vi "Erase and Write pulse control V1.1.vi"() -> ()   [LabVIEW 2016]
uses:
  <userlib>/LevyLab/Relay Box/Type_defs/Resistor--enum.ctl
panel:
  out "error out":errorcluster
  in  "error in":errorcluster
  in  "Set Resistance":T1=enum."1G ohm"
  in  "Z SetPoint: Lift the tip a little":dbl=-0.03 format="%#_6p"
  in  "Withdraw tip?":bool
  in  "wait time second pulse 3":u32=500
  in  "Second pulse 3":dbl=16.0 format="%_5p"
  in  "wait time between 3":u32=500
  in  "Wait time first pulse  2":u32=2000
  in  "First pulse 3":dbl=-15.0 format="%_5p"
  in  "Z SetPoint 3":dbl=-0.29 format="%#_6p"
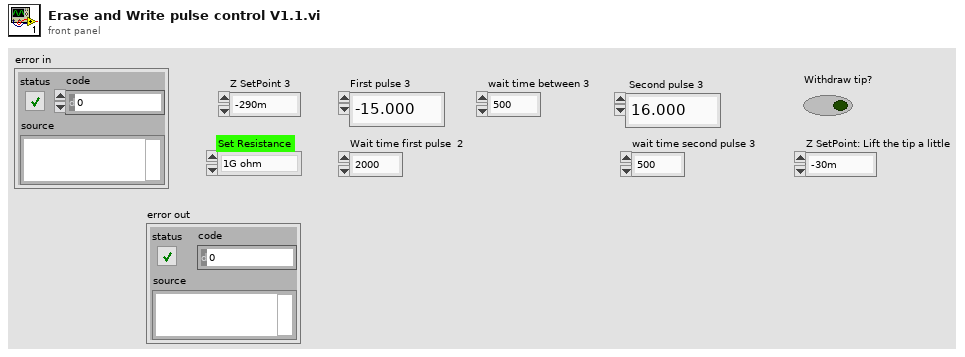
[diagram p1: front panel]
types:
  T1 = typedef "Resistor--enum.ctl" = enum16{"open", "discharge tip", "0 ohms", "100k ohm", "10M ohm", "1G ohm"}
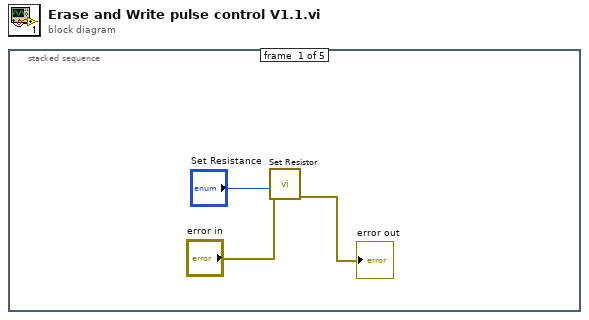
[diagram p0: block diagram]
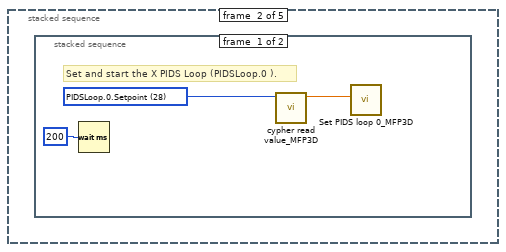
[diagram p2: hidden frame]
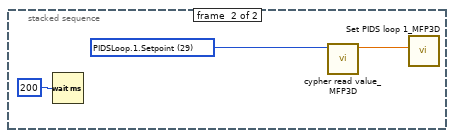
[diagram p3: hidden frame]
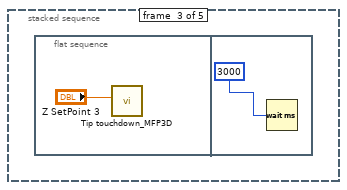
[diagram p4: hidden frame]
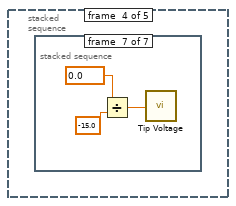
[diagram p5: hidden frame]
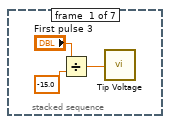
[diagram p6: hidden frame]
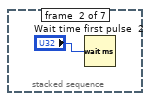
[diagram p7: hidden frame]
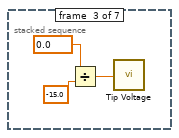
[diagram p8: hidden frame]
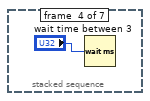
[diagram p9: hidden frame]
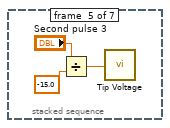
[diagram p10: hidden frame]
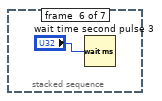
[diagram p11: hidden frame]
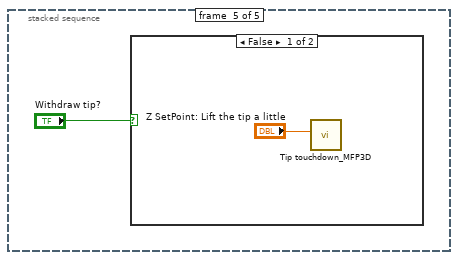
[diagram p12: hidden frame]
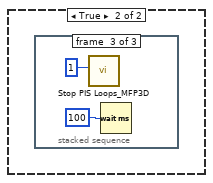
[diagram p13: hidden frame]
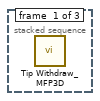
[diagram p14: hidden frame]
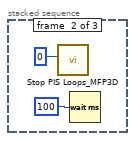
[diagram p15: hidden frame]
diagram:
  n1 = stacked-sequence {
    frame #0 {
      n2 = call <userlib>:"Set Resistor.vi"("error in"="error in", "Set Resistance"="Set Resistance") -> ("error out"=→"error out":errorcluster)  [unwired: 9 in]
    }
    frame #1 {
      n3 = stacked-sequence {
        frame #0 {
          w5 = u16 28 items=["XSensor", "YSensor", "ZSensor", "InA", "InB", "InFast", "In_Amplitude1", "In_Amplitude2", "In_Phase1", "In_Phase2", "PiezoX", "PiezoY", "PiezoZ", "OutA", "OutB", "OutC", "DDS_Frequency1", "DDS_Frequency2", "DDS_Amplitude1", "DDS_Amplitude2", "DDS_DCOffset", "Laser_Sum", "Laser_Difference", "Laser_Lateral", "XLVDT Sensitivity", "YLVDT Sensitivity", "XLVDT Offset", "YLVDT Offset", "PIDSLoop.0.Setpoint", "PIDSLoop.1.Setpoint"] ("Input")
          # "Set and start the X PIDS Loop (PIDSLoop.0 )."
          n4 = Wait (ms)(milliseconds to wait=u32 200) -> ()  [unwired: 1 out]
          n5 = call <vilib>:"cypher read value_MFP3D.vi"("Input"=w5) -> ("Result"=w6:dbl)  [unwired: 10 in]
          n6 = call <vilib>:"Set PIDS loop 0_MFP3D.vi"("X  Setpoint"=w6) -> ()  [unwired: 11 in]
        }
        frame #1 {
          w8 = u16 29 items=["XSensor", "YSensor", "ZSensor", "InA", "InB", "InFast", "In_Amplitude1", "In_Amplitude2", "In_Phase1", "In_Phase2", "PiezoX", "PiezoY", "PiezoZ", "OutA", "OutB", "OutC", "DDS_Frequency1", "DDS_Frequency2", "DDS_Amplitude1", "DDS_Amplitude2", "DDS_DCOffset", "Laser_Sum", "Laser_Difference", "Laser_Lateral", "XLVDT Sensitivity", "YLVDT Sensitivity", "XLVDT Offset", "YLVDT Offset", "PIDSLoop.0.Setpoint", "PIDSLoop.1.Setpoint"] ("Input")
          n7 = Wait (ms)(milliseconds to wait=u32 200) -> ()  [unwired: 1 out]
          n8 = call <vilib>:"cypher read value_MFP3D.vi"("Input"=w8) -> ("Result"=w7:dbl)  [unwired: 10 in]
          n9 = call <vilib>:"Set PIDS loop 1_MFP3D.vi"("Y Setpoint"=w7) -> ()  [unwired: 11 in]
        }
      }
    }
    frame #2 {
      n10 = flat-sequence {
        frame #0 {
          n11 = call <vilib>:"Tip touchdown_MFP3D.vi"("Z SetPoint"="Z SetPoint 3") -> ()  [unwired: 11 out]
        }
        frame #1 {
          n12 = Wait (ms)(milliseconds to wait=u32 3000 ("Wait time first pulse  2")) -> ()  [unwired: 1 out]
        }
      }
    }
    frame #3 {
      n13 = stacked-sequence {
        frame #0 {
          n14 = Divide(x="First pulse 3", y=-15.0) -> (x/y=w12:dbl)
          n15 = call <userlib>:"Tip Voltage.vi"("Output Voltage"=w12) -> ()  [unwired: 1 out]
        }
        frame #1 {
          n16 = Wait (ms)(milliseconds to wait="Wait time first pulse  2") -> ()  [unwired: 1 out]
        }
        frame #2 {
          n17 = Divide(x=0.0 ("Output Voltage 2"), y=-15.0) -> (x/y=w18:dbl)
          n18 = call <userlib>:"Tip Voltage.vi"("Output Voltage"=w18) -> ()  [unwired: 1 out]
        }
        frame #3 {
          n19 = Wait (ms)(milliseconds to wait="wait time between 3") -> ()  [unwired: 1 out]
        }
        frame #4 {
          n20 = Divide(x="Second pulse 3", y=-15.0) -> (x/y=w22:dbl)
          n21 = call <userlib>:"Tip Voltage.vi"("Output Voltage"=w22) -> ()  [unwired: 1 out]
        }
        frame #5 {
          n22 = Wait (ms)(milliseconds to wait="wait time second pulse 3") -> ()  [unwired: 1 out]
        }
        frame #6 {
          n23 = Divide(x=0.0 ("Output Voltage 2"), y=-15.0) -> (x/y=w26:dbl)
          n24 = call <userlib>:"Tip Voltage.vi"("Output Voltage"=w26) -> ()  [unwired: 1 out]
        }
      }
    }
    frame #4 {
      n25 = case shown="False" "Withdraw tip?" {
        frame False {
          n26 = call <vilib>:"Tip touchdown_MFP3D.vi"("Z SetPoint"="Z SetPoint: Lift the tip a little") -> ()  [unwired: 11 out]
        }
        frame True {
          n27 = stacked-sequence {
            frame #0 {
              n28 = call <vilib>:"Tip Withdraw_MFP3D.vi"() -> ()  [unwired: 1 in]
            }
            frame #1 {
              n29 = call <vilib>:"Stop PIS Loops_MFP3D.vi"("PIS Loop Number (0-5)"=u32 0) -> ()  [unwired: 11 out]
              n30 = Wait (ms)(milliseconds to wait=u32 100) -> ()  [unwired: 1 out]
            }
            frame #2 {
              n31 = call <vilib>:"Stop PIS Loops_MFP3D.vi"("PIS Loop Number (0-5)"=u32 1) -> ()  [unwired: 11 out]
              n32 = Wait (ms)(milliseconds to wait=u32 100) -> ()  [unwired: 1 out]
            }
          }
        }
      }
    }
  }
